vi "Math-Zero Pad.vi"(0 "Signal":dbl[](array[numeric]), 5 "Resol (Hz)":dbl, 7 "Fs (Hz)":dbl, 11 "Window":bool) -> (4 "Zero-padded signal":dbl[](array[numeric]), 8 "Scale factor":dbl)   [LabVIEW 2020]
uses:
  <vilib>/Analysis/4window.llb/Hamming Window (DBL).vi
  <vilib>/Analysis/4window.llb/AllCosWindow (DBL).vi
  <vilib>/Analysis/NI_AALPro.lvlib
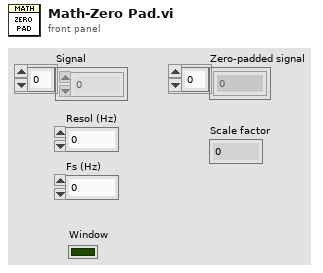
[diagram p1: front panel]
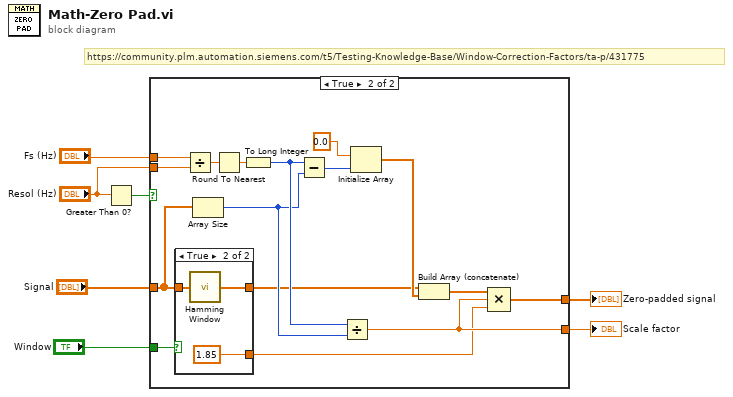
[diagram p0: block diagram]
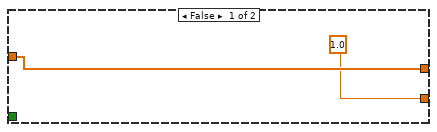
[diagram p2: hidden frame]
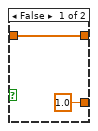
[diagram p3: hidden frame]
diagram:
  # "https://community.plm.automation.siemens.com/t5/Testing-Knowledge-Base/Window-Correction-Factors/ta-p/431775"
  n1 = Greater Than 0?(x="Resol (Hz)") -> (x > 0?=w2:bool)
  n2 = case shown="True" w2 {
    tunnel: "Fs (Hz)" -> [_ w25]
    tunnel: "Resol (Hz)" -> [_ w24]
    tunnel: "Signal" -> [w9 w20]
    tunnel: [w9 w16] -> w5
    tunnel: [1.0 w15] -> w4
    tunnel: "Window" -> [_ w10]
    frame False {
    }
    frame True {
      n3 = case shown="True" w10 {
        tunnel: w20 -> [w27 w30]
        tunnel: [w27 w29] -> w12
        tunnel: [1.0 1.85] -> w11
        frame False {
        }
        frame True {
          n4 = call-poly <vilib>:"Hamming Window.vi"("X"=w30) -> ("Windowed X"=w29:dbl[])  [unwired: 1 out]
        }
      }
      n5 = Divide(x=w25, y=w24) -> (x/y=w23:dbl)
      n6 = Array Size(array=w20) -> (size(s)=w13:i32)
      n7 = Round To Nearest(number=w23) -> (nearest integer value=w22:dbl)
      n8 = To Long Integer(number=w22) -> (32bit integer=w14:i32)
      n9 = Subtract(x=w14, y=w13) -> (x-y=w17:i32)
      n10 = Divide(x=w14, y=w13) -> (x/y=w15:dbl)
      n11 = Initialize Array(0.0, w17) -> (w19:dbl[])
      n12 = Build Array (concatenate)(w12, w19) -> (w18:dbl[])
      n13 = Compound Arithmetic op=MULTIPLY(w18, w15, w11) -> (w16:dbl[])
    }
  }
  "Scale factor" <- w4
  "Zero-padded signal" <- w5
